vi "Set Class Reference.vi"(8 "error in (no error)":errorcluster, 10 "LabVIEW Class":refnum<vi>, 11 "Class Reference Control in":refnum<class "Class Reference Control.lvclass">) -> (0 "error out":errorcluster, 3 "Class Reference Control out":refnum<class "Class Reference Control.lvclass">)   [LabVIEW 2016, in "Class Reference Control.lvclass"]
uses:
  Class Reference Control.lvclass
  C:/Users/tblair/Documents/Git Projects/Drag and Drop VI Tool/Reference Control/Reference Control.lvclass
  Class Reference Control.lvclass/Class Reference Control.ctl
  Reference Control/Reference Control.lvclass
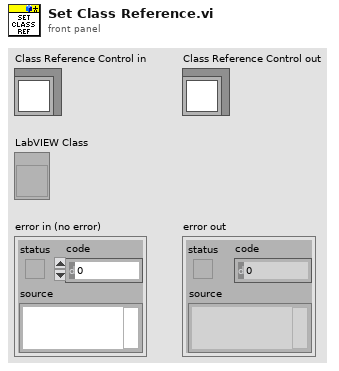
[diagram p1: front panel]
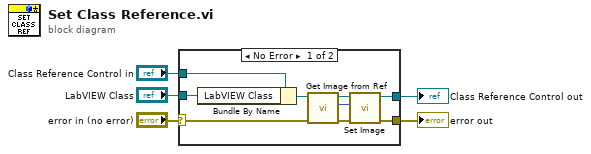
[diagram p0: block diagram]
diagram:
  n1 = case shown="No Error" "error in (no error)" {
    selector: "error in (no error)" -> [w9 w16]
    tunnel: [w7 w16] -> w4
    tunnel: [w10 w15] -> w2
    tunnel: "Class Reference Control in" -> [w14 w15]
    tunnel: "LabVIEW Class" -> [w13 _]
    frame No Error {
      n2 = Bundle By Name(cluster=w14, "LabVIEW Class"=w13) -> (w12:refnum<class "Class Reference Control.lvclass">)
      n3 = call-dynamic "Get Image from Ref.vi"("error in (no error)"=w9, "Class Reference Control in"=w12) -> ("error out"=w8:errorcluster, "new picture"=w6:picture, "Class Reference Control out"=w11:refnum<class "Class Reference Control.lvclass">)  [unwired: 7 in]
      n4 = call "Set Image.vi"("error in (no error)"=w8, "Picture"=w6, "Reference Control in"=w11) -> ("error out"=w7:errorcluster, "Reference Control out"=w10:refnum<class "Class Reference Control.lvclass">)  [unwired: 7 in]
    }
    frame Error {
    }
  }
  "error out" <- w4
  "Class Reference Control out" <- w2
